vi "Tracepoint_ServerConnection.vi"(8 "error in (no error)":errorcluster, 9 "URL":string, 11 "Qbus":refnum<class "Qbus.lvclass">) -> (0 "error out":errorcluster)   [LabVIEW 2017, in "OPCUAClient.lvlib"]
uses:
  <vilib>/addons/InsightCM/Devices/Shared/Common/OPCUAClient/OPCUAClient.lvlib
  <vilib>/addons/Qbus/Qbus.lvclass
  <vilib>/addons/TraceLogger/TraceLogger.lvlib
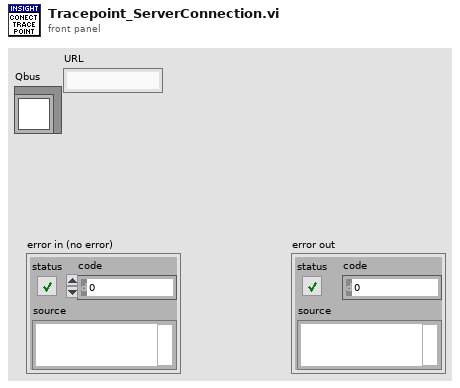
[diagram p1: front panel]
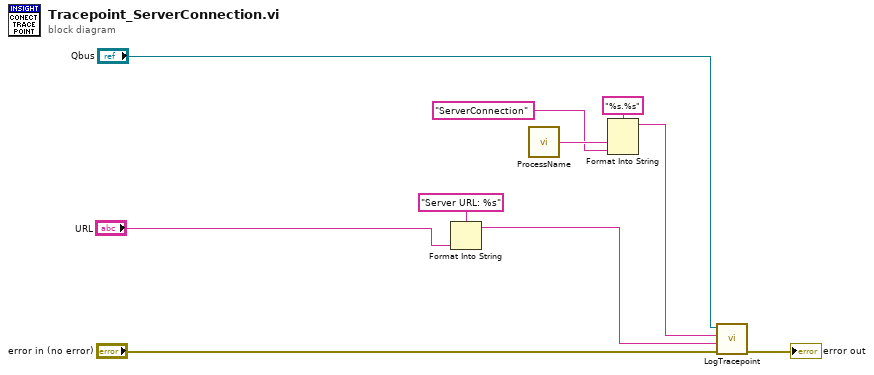
[diagram p0: block diagram]
diagram:
  n1 = Format Into String(format string="Server URL: %s", "URL") -> (resulting string=w5:string)  [unwired: 2 in, 1 out]
  n2 = call <vilib>:"ProcessName.vi"() -> ("process name"=w7:string)  [unwired: 5 in]
  n3 = Format Into String(format string="%s.%s", w7, "ServerConnection" ("tracepoint")) -> (resulting string=w6:string)  [unwired: 2 in, 1 out]
  n4 = call <vilib>:"LogTracepoint.vi"("error in (no error)"="error in (no error)", "log string"=w5, "tracepoint"=w6, "qbus in"="Qbus") -> ("error out"=→"error out":errorcluster)  [unwired: 6 in, 1 out]
